vi "always includes.vi"   [LabVIEW 2013, in "configuration library.lvlib"]
uses:
  configuration library.lvlib
  <vilib>/NI/Tag Bus Module Framework/module configuration/TBM module configuration.lvclass
  <vilib>/NI/Tag Bus Module Framework/channel/TBM channel.lvclass
  <vilib>/CEF_TreeControl/Node/NISE_CEF_Node.lvclass
  <vilib>/NI/Module Execution Interface/Engine Configuration/engine configuration.lvclass
  Framework Configuration Classes/system configuration/PL_System Configuration.lvclass
  <vilib>/CEF_TreeControl/Repository/NISE_CEF_Repository.lvclass
  Configuration Editor/Classes/Engine Parent/Engine Parent Editor Node.lvclass
  Configuration Editor/Classes/Targets/Targets.lvclass
  Configuration Editor/Classes/SystemConfigRepo/SystemConfigRepo.lvclass
  Framework Configuration Classes/target configuration/PL_Target Configuration.lvclass
  <vilib>/NI/Tag Bus Module Framework/root configuration/TBM configuration.lvclass
  Configuration Editor/Classes/TBM Configuration Node/TBM Configuration Node.lvclass
  <vilib>/NI/Module Timing Source/timing source/TBM timing source.lvclass
  Configuration Editor/Classes/Systems/Systems.lvclass
  Configuration Editor/Classes/EngineTags/EngineTags.lvclass
  Configuration Editor/Classes/Module editor node/module editor node.lvclass
  Configuration Editor/subVIs/Add status to name.vi
  Configuration Editor/subVIs/Glyphs Status.ctl
  Configuration Editor/PL Framework Configuration Tool.lvlib
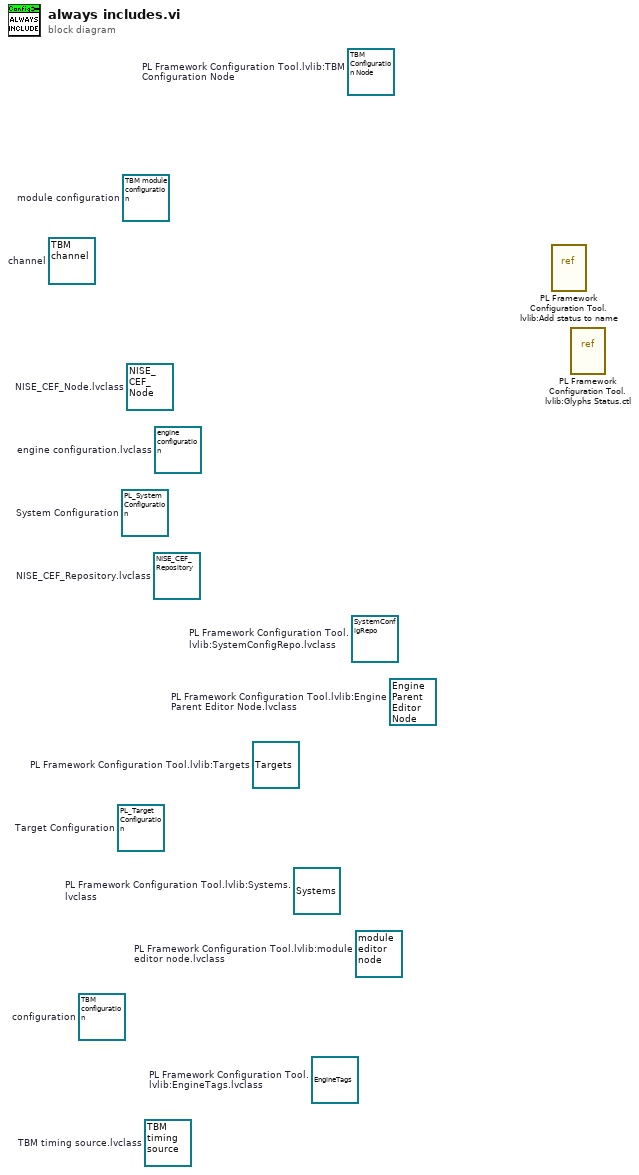
[diagram p0: block diagram]
diagram:
  (unwired) refnum<class "module editor node.lvclass"> refnum  # PL Framework Configuration Tool.lvlib:module editor node.lvclass
  (unwired) refnum<class "EngineTags.lvclass"> refnum  # PL Framework Configuration Tool.lvlib:EngineTags.lvclass
  (unwired) refnum<class "Systems.lvclass"> refnum  # PL Framework Configuration Tool.lvlib:Systems.lvclass
  (unwired) refnum<class "TBM timing source.lvclass"> refnum  # TBM timing source.lvclass
  (unwired) refnum<class "TBM Configuration Node.lvclass"> refnum  # PL Framework Configuration Tool.lvlib:TBM Configuration Node
  (unwired) refnum<class "TBM configuration.lvclass"> refnum  # configuration
  (unwired) refnum<class "PL_Target Configuration.lvclass"> refnum  # Target Configuration
  (unwired) refnum<class "SystemConfigRepo.lvclass"> refnum  # PL Framework Configuration Tool.lvlib:SystemConfigRepo.lvclass
  (unwired) refnum<class "Targets.lvclass"> refnum  # PL Framework Configuration Tool.lvlib:Targets
  (unwired) refnum<class "Engine Parent Editor Node.lvclass"> refnum  # PL Framework Configuration Tool.lvlib:Engine Parent Editor Node.lvclass
  (unwired) refnum<class "NISE_CEF_Repository.lvclass"> refnum  # NISE_CEF_Repository.lvclass
  (unwired) refnum<class "PL_System Configuration.lvclass"> refnum  # System Configuration
  (unwired) refnum<class "engine configuration.lvclass"> refnum  # engine configuration.lvclass
  (unwired) refnum<class "NISE_CEF_Node.lvclass"> refnum  # NISE_CEF_Node.lvclass
  (unwired) refnum<class "TBM channel.lvclass"> refnum  # channel
  (unwired) refnum<class "TBM module configuration.lvclass"> refnum  # module configuration
  n1 = vi-ref "PL Framework Configuration Tool.lvlib:Add status to name.vi"() -> ()  [unwired: 1 out]
  n2 = vi-ref "PL Framework Configuration Tool.lvlib:Glyphs Status.ctl"() -> ()  [unwired: 1 out]
